vi "Test 4 Go Around.vi"(8 "error in (no error)":errorcluster, 11 "Test Case In":refnum<class "Tests.lvclass">) -> (0 "error out":errorcluster, 3 "Test Case Out":refnum<class "Tests.lvclass">)   [LabVIEW 2021, in "Tests.lvclass"]
uses:
  Tests.lvclass
  C:/Program Files (x86)/National Instruments/LabVIEW 2021/vi.lib/Astemes/LUnit/Test Case.lvclass
  <vilib>/Astemes/LUnit/Test Case.lvclass/Test Case.ctl
  4993e8ee-a06a-463a-9684-69129f64d5ce.vi
  <vilib>/Astemes/LUnit/Append Pass Result.vi
  <vilib>/Astemes/LUnit/Append Fail Result.vi
  <vilib>/Astemes/LUnit/Describe Comparison.vi
  <vilib>/Astemes/LUnit/Compare Variants.vi
  <vilib>/Astemes/LUnit/Variant to string.vi
  <vilib>/Utility/Data Type/Get Type Information.vi
  <vilib>/Utility/LVClass/Get LV Class Name.vi
  Proto/Proto.lvclass
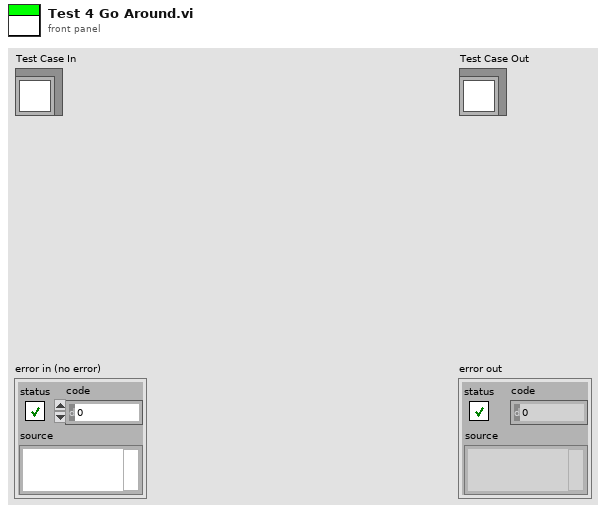
[diagram p1: front panel]
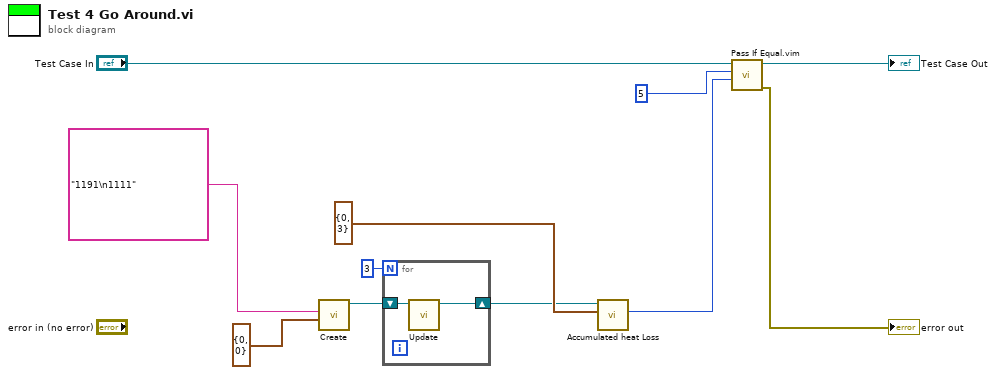
[diagram p0: block diagram]
diagram:
  n1 = call "Create.vi"("Start Position"=cluster{"Row":i32, "Col":i32} {"Row"=0, "Col"=0}, "Input"="1191\n1111") -> ("Proto"=w8:refnum<class "Proto.lvclass">)  [unwired: 9 in]
  n2 = for {
    N: 3 -> [_]
    shift-right: [w12] -> w2
    shift-left: w8 -> [w13]
    n3 = call "Update.vi"("Proto in"=w13) -> ("Proto out"=w12:refnum<class "Proto.lvclass">)  [unwired: 9 in, 1 out]
  }
  n4 = call "Accumulated heat Loss.vi"("Coord"=cluster{"Row":i32, "Col":i32} {"Row"=0, "Col"=3}, "Proto in"=w2) -> ("Min Heat"=w5:i32)  [unwired: 8 in, 1 out]
  n5 = call "Pass If Equal.vim"("Actual"=w5, "Expected"=5 ("Heat"), "LUnit Test Case In"="Test Case In") -> ("error out"=→"error out":errorcluster, "LUnit Test Case Out"=→"Test Case Out":refnum<class "Tests.lvclass">)  [unwired: 7 in]
